vi "Initialize Main Page.vi"(8 "error in (no error)":errorcluster, 10 "Main Page Controls":T3, 11 "Item Ref in":T2 format="%.0x") -> (0 "error out":errorcluster, 3 "Item Ref out":T2 format="%.0x")   [LabVIEW 2020, in "NI-SWITCH System Explorer.lvlib"]
uses:
  NI-SWITCH System Explorer.lvlib
  Main Page Controls.ctl
  <vilib>/NI VeriStand/Custom Device API/Custom Device Item Ref.ctl
  <instrlib>/niSwitch/niSwitch.llb/niSwitch Topologies.ctl
  Scripting/NI-SWITCH Scripting.lvlib
  <vilib>/NI VeriStand/Custom Device API/Custom Device API.lvlib
panel:
  in  "topology name":T1="Configured Topology"
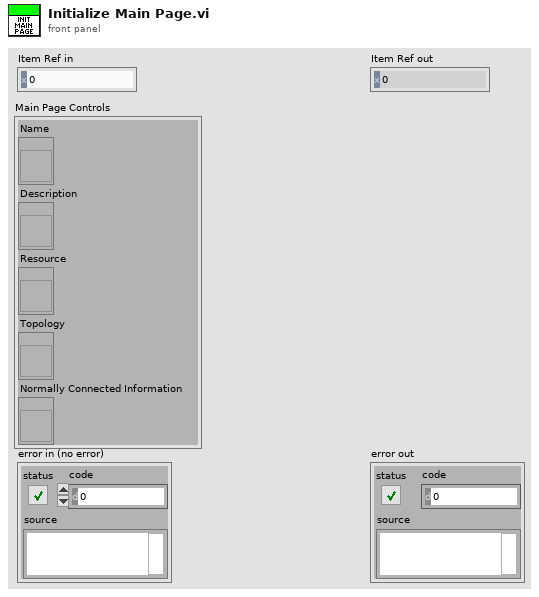
[diagram p1: front panel]
types:
  T1 = typedef "niSwitch Topologies.ctl" = string
  T2 = typedef "Custom Device API.lvlib/Custom Device Item Ref.ctl" = u64
  T3 = typedef "NI-SWITCH System Explorer.lvlib/Main Page Controls.ctl" = cluster{"Name":refnum<vi>, "Description":refnum<vi>, "Resource":refnum<vi>, "Topology":refnum<vi>, "Normally Connected Information":refnum<vi>}
  T4 = typedef "NI-SWITCH Scripting.lvlib/NI-SWITCH All Properties.ctl" = cluster{"Resource":string, "Topology":string, "Description":string}
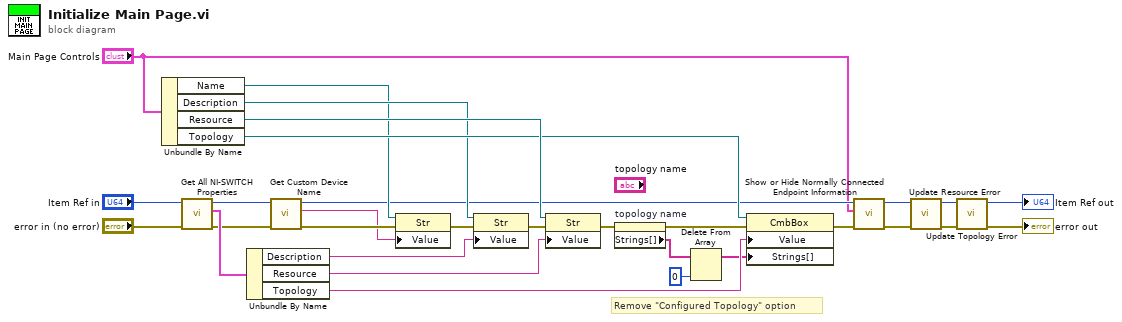
[diagram p0: block diagram]
diagram:
  # "Remove \"Configured Topology\" option"
  n1 = Unbundle By Name("Main Page Controls") -> ("Name"=w11:refnum<vi>, "Description"=w24:refnum<vi>, "Resource"=w30:refnum<vi>, "Topology"=w26:refnum<vi>)
  n2 = call "Get All NI-SWITCH Properties.vi"("error in"="error in (no error)", "ni-switch custom device in"="Item Ref in") -> ("error out"=w20:errorcluster, "properties"=w29:T4, "ni-switch custom device out"=w12:T2)  [unwired: 7 in]
  n3 = Unbundle By Name(w29) -> ("Description"=w23:string, "Resource"=w28:string, "Topology"=w27:string)
  n4 = call "Get Custom Device Name.vi"("error in"=w20, "ni-switch custom device in"=w12) -> ("error out"=w13:errorcluster, "name"=w10:string, "ni-switch custom device out"=w8:T2)  [unwired: 7 in]
  n5 = property class="Str"(reference=w11, error in=w13, "Value"=w10) -> (error out=w14:errorcluster)  [unwired: 1 out]
  n6 = property class="Str"(reference=w24, error in=w14, "Value"=w23) -> (error out=w25:errorcluster)  [unwired: 1 out]
  n7 = property class="Str"(reference=w30, error in=w25, "Value"=w28) -> (error out=w19:errorcluster)  [unwired: 1 out]
  n8 = property on="topology name" class="CmbBox (strict)"(error in=w19) -> (error out=w18:errorcluster, "Strings[]"=w17:string[])  [unwired: 1 in, 1 out]
  n9 = Delete From Array(array=w17, index=0) -> (array with subset deleted=w16:string[])  [unwired: 1 in, 1 out]
  n10 = property class="CmbBox"(reference=w26, error in=w18, "Value"=w27, "Strings[]"=w16) -> (error out=w9:errorcluster)  [unwired: 1 out]
  n11 = call "Show or Hide Normally Connected Endpoint Information.vi"("error in (no error)"=w9, "Main Page Controls"="Main Page Controls", "ni-switch custom device in"=w8) -> ("error out"=w6:errorcluster, "ni-switch custom device out"=w4:T2)  [unwired: 7 in]
  n12 = call "Update Resource Error.vi"("error in"=w6, "ni-switch custom device in"=w4) -> ("error out"=w5:errorcluster, "ni-switch custom device out"=w2:T2)  [unwired: 8 in]
  n13 = call "Update Topology Error.vi"("error in"=w5, "ni-switch custom device in"=w2) -> ("error out"=→"error out":errorcluster, "ni-switch custom device out"=→"Item Ref out":T2)  [unwired: 8 in]
